vi "main.vi"() -> ()   [LabVIEW 2021]
uses:
  <vilib>/Instr/_visa.llb/VISA Configure Serial Port (Instr).vi
  lib/EMGParser.dll
panel:
  out "mag":i32[](array[numeric])
  out "temperature":sgl
  out "spo2":sgl[](array[numeric])
  out "emgRaw":i32
  out "acc":sgl[](array[numeric])
  in  "停止":bool
  in  "VISA resource name":refnum<visa-resource-name> caption="VISA资源名称"
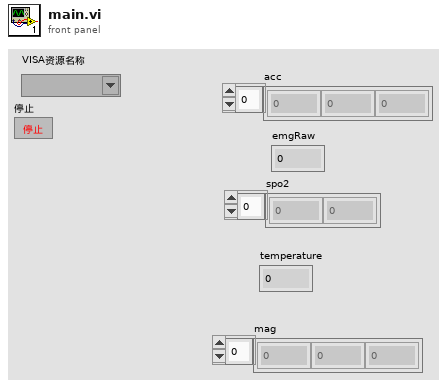
[diagram p1: front panel]
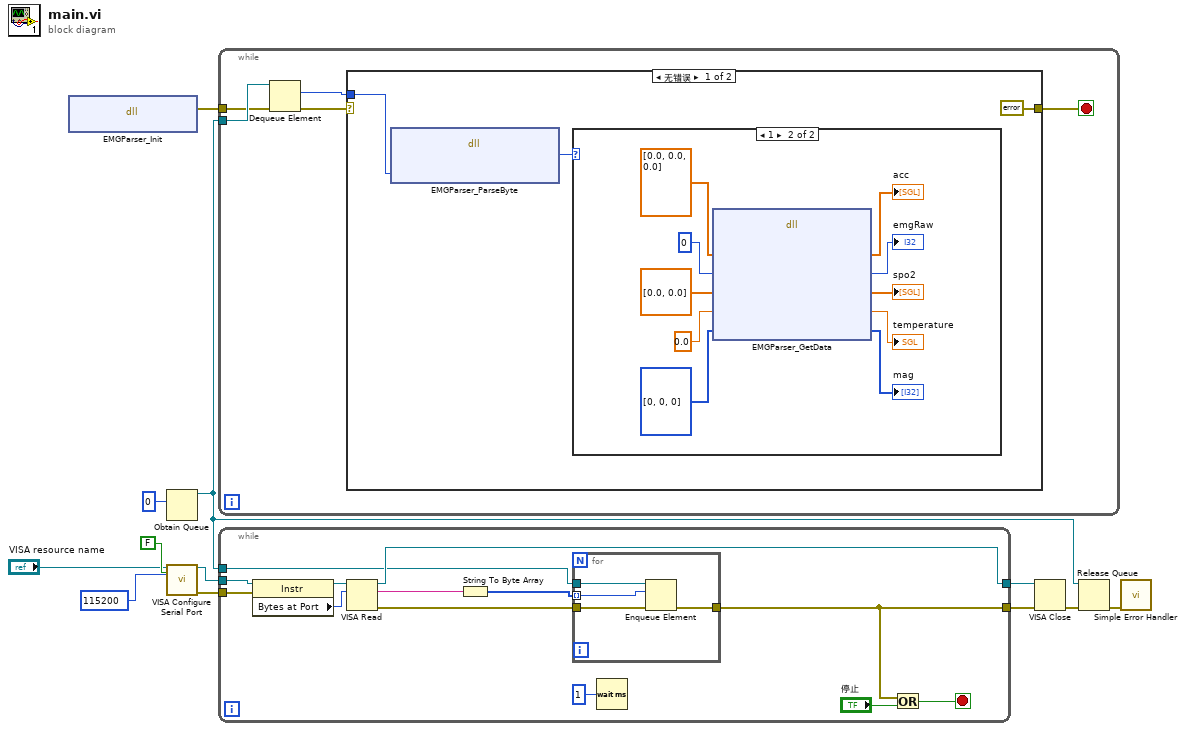
[diagram p0: block diagram]
diagram:
  n1 = dll-call lib="D:/labview/EMGParser/lib/EMGParser.dll" fn="EMGParser_Init"() -> (error out=w1:errorcluster)  [unwired: 4 in, 1 out]
  n2 = Obtain Queue(element data type=u8 0) -> (queue out=w2:refnum<queue>)  [unwired: 4 in, 2 out]
  n3 = call-poly "VISA Configure Serial Port"("VISA resource name"="VISA resource name", "Enable Termination\nChar (T)"=FALSE ("Enable Termination\nChar (T)"), "baud rate (9600)"=u32 115200) -> ("VISA resource name out"=w8:refnum<visa-resource-name>, "error out"=w7:errorcluster)  [unwired: 11 in]
  n4 = while {
    tunnel: w2 -> [w17]
    tunnel: w1 -> [w15]
    stop <- w14 stop-if-true
    n5 = Dequeue Element(queue=w17, error in (no error)=w15) -> (element=w13:u8, error out=w16:errorcluster)  [unwired: 1 in, 2 out]
    n6 = case shown="无错误" w16 {
      selector: w16 -> [_ w31]
      tunnel: [errorcluster {"status"=FALSE, "code"=0, "source"=""} ("error IO") w31] -> w14
      tunnel: w13 -> [w19 _]
      frame No Error {
        n7 = dll-call lib="D:/labview/EMGParser/lib/EMGParser.dll" fn="EMGParser_ParseByte"("b"=w19) -> ("返回类型"=w18:i32)  [unwired: 4 in, 2 out]
        n8 = case shown="1" w18 {
          frame 0, Default {
          }
          frame 1 {
            n9 = dll-call lib="D:/labview/EMGParser/lib/EMGParser.dll" fn="EMGParser_GetData"("acc"=sgl[] [0.0, 0.0, 0.0], "emgRaw"=0, "spo2"=sgl[] [0.0, 0.0], "temperature"=sgl 0.0, "mag"=i32[] [0, 0, 0]) -> ("acc"=→"acc":sgl[], "emgRaw"=→"emgRaw":i32, "spo2"=→"spo2":sgl[], "temperature"=→"temperature":sgl, "mag"=→"mag":i32[])  [unwired: 4 in, 2 out]
          }
        }
      }
      frame Error {
      }
    }
  }
  n10 = while {
    tunnel: [w44] -> w9
    tunnel: w8 -> [w43]
    tunnel: w7 -> [w42]
    tunnel: w2 -> [w37]
    tunnel: [w33] -> w5
    stop <- w32 stop-if-true
    n11 = property class="Instr"(reference=w43, error in=w42) -> (reference out=w41:refnum<visa-resource-name>, "Bytes at Port"=w40:u32)  [unwired: 1 out]
    n12 = VISA Read(VISA resource name=w41, byte count=w40) -> (VISA resource name out=w44:refnum<visa-resource-name>, read buffer=w38:string, error out=w35:errorcluster)  [unwired: 1 in, 1 out]
    n13 = String To Byte Array(string=w38) -> (unsigned byte array=w36:u8[])
    n14 = for {
      tunnel: w37 -> [w48]
      tunnel: w36 -> [w47] mode=indexing
      tunnel: w35 -> [w46]
      tunnel: [w45] -> w33
      n15 = Enqueue Element(queue=w48, element=w47, error in (no error)=w46) -> (error out=w45:errorcluster)  [unwired: 1 in, 2 out]
    }
    n16 = Wait (ms)(milliseconds to wait=u32 1 ("等待时间（毫秒）")) -> ()  [unwired: 1 out]
    n17 = Or(x=w33, y="停止") -> (x .or. y?=w32:bool)
  }
  n18 = VISA Close(VISA resource name=w9, error in (no error)=w5) -> (error out=w4:errorcluster)
  n19 = Release Queue(queue=w2, error in (no error)=w4) -> (error out=w3:errorcluster)  [unwired: 1 in, 2 out]
  n20 = call <vilib>:"Simple Error Handler.vi"("error in (no error)"=w3) -> ()  [unwired: 4 in, 5 out]
